vi "Read Module Menu Name.vi"(8 "error in":errorcluster, 11 "fixed channel editor in":refnum<class "fixed channel editor.lvclass">) -> (0 "error out":errorcluster, 2 "Menu Name":string, 3 "fixed channel editor out":refnum<class "fixed channel editor.lvclass">)   [LabVIEW 2013, in "fixed channel editor.lvclass"]
uses:
  fixed channel editor.lvclass
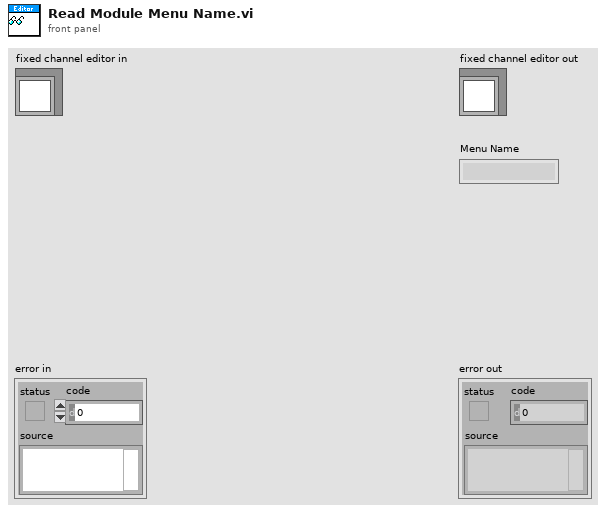
[diagram p1: front panel]
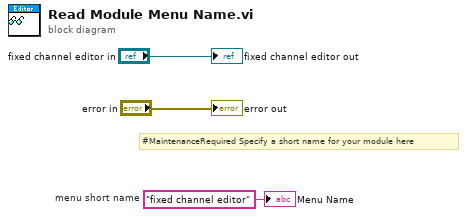
[diagram p0: block diagram]
diagram:
  w1 = "fixed channel editor"  # menu short name
  # "#MaintenanceRequired Specify a short name for your module here"
  "error out" <- "error in"
  "fixed channel editor out" <- "fixed channel editor in"
  "Menu Name" <- w1
